vi "GEvt-Generate with Rule Check.vi"(7 "LogFilter In":refnum<class "LogFilter.lvclass">, 10 "Event Data":T2, 11 "CSM Global Log Event In":T1) -> (3 "CSM Global Log Event Out":T1)   [LabVIEW 2017, in "Communicable State Machine.lvlib"]
doc: "### GEvt-Generate with Rule Check.vi\n\n-- <b>Controls</b> --\n- <b>LogFilter in</b>:\n- <b>event data</b>:\n- <b>CSM Global Log Event in</b>:\n\n-- <b>Indicators</b> --\n- <b>CSM Global Log Event out</b>:"
uses:
  Communicable State Machine.lvlib
  Typedef/_CSM_GlobalLog_MSG.ctl
  Typedef/_CSM_Response Source Message.ctl
  Typedef/_CSM_GlobalLog_MSG_TYPE.ctl
  LogFilter/LogFilter.lvclass
  GEvt-Refs.ctl
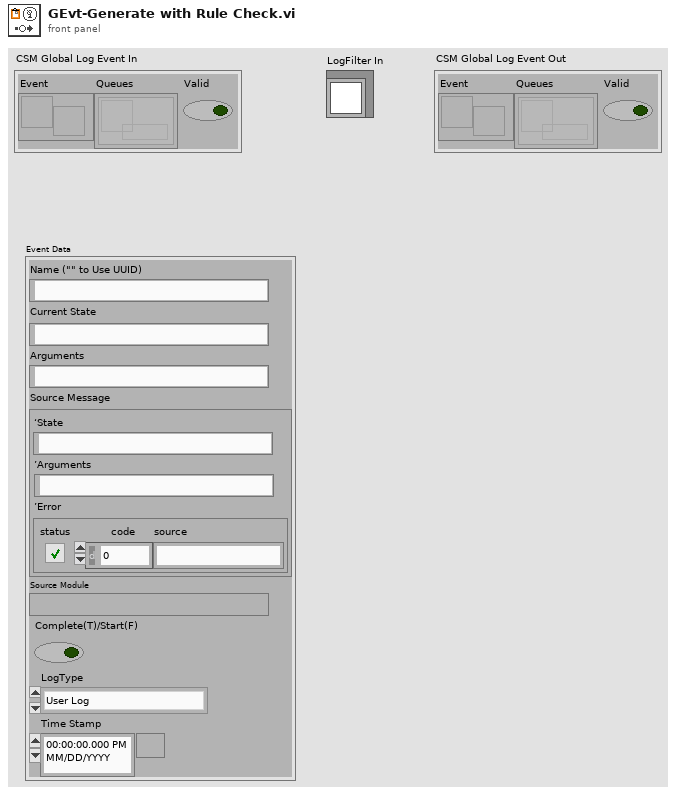
[diagram p1: front panel]
types:
  T1 = typedef "Communicable State Machine.lvlib/GEvt-Refs.ctl" = cluster{"Event":refnum<user-event>, "Queues":refnum<queue>[], "Valid":bool}
  T2 = typedef "Communicable State Machine.lvlib/_CSM_GlobalLog_MSG.ctl" = cluster{"Name (\"\" to Use UUID)":string, "Current State":string, "Arguments":string, "Source Message":T3, "Source Module":string, "Complete(T)/Start(F)":bool, "LogType":T4, "Time Stamp":timestamp}
  T3 = typedef "Communicable State Machine.lvlib/_CSM_Response Source Message.ctl" = cluster{"‘State":string, "’Arguments":string, "’Error":errorcluster}
  T4 = typedef "Communicable State Machine.lvlib/_CSM_GlobalLog_MSG_TYPE.ctl" = enum16{"User Log", "State Change", "Status", "Interrupt", "Register", "Unregister", "Error Log", "Module Created", "Module Destroyed", "Async Message", "No-Rep Async Message", "Sync Message"}
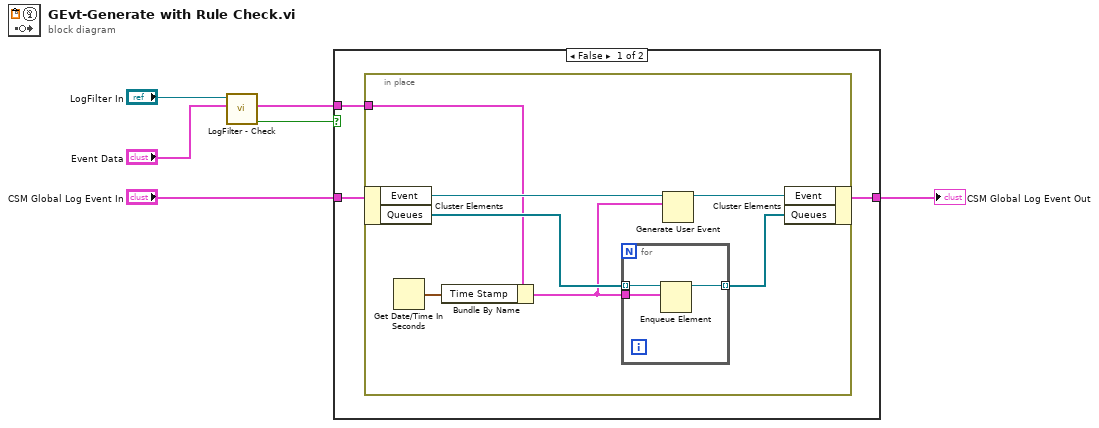
[diagram p0: block diagram]
diagram:
  n1 = call "LogFilter - Check.vi"("Cross CSM Data In"="Event Data", "GlobalLogFilter In"="LogFilter In") -> ("Matched? (Dup)"=w6:bool, "Cross CSM Data Out"=w5:T2)  [unwired: 7 in, 1 out]
  n2 = case shown="False" w6 {
    tunnel: "CSM Global Log Event In" -> [w8 w20]
    tunnel: [w7 w20] -> w2
    tunnel: w5 -> [w9 _]
    frame False {
      n3 = in-place {
        in-place-border: w9 -> [w12]
        n4 = in-place-cluster #1(w8) -> ("Event"=w16:refnum<user-event>, "Queues"=w14:refnum<queue>[])
        n5 = Get Date/Time In Seconds() -> (seconds since 1Jan1904=w10:timestamp)
        n6 = Bundle By Name(cluster=w12, "Time Stamp"=w10) -> (w11:T2)
        n7 = for {
          tunnel: w14 -> [w19] mode=indexing
          tunnel: [w18] -> w13 mode=indexing
          tunnel: w11 -> [w17]
          n8 = Enqueue Element(queue=w19, element=w17) -> (queue out=w18:refnum<queue>)  [unwired: 2 in, 2 out]
        }
        n9 = Generate User Event(user event=w16, event data cluster=w11) -> (user event out=w15:refnum<user-event>)  [unwired: 2 in, 1 out]
        n10 = in-place-cluster #1("Event"=w15, "Queues"=w13) -> (w7:T1)
      }
    }
    frame True {
    }
  }
  "CSM Global Log Event Out" <- w2
